vi "nominal dataset create.vi"(7 "out_dataset":i32, 8 "error in (no error)":errorcluster, 9 "description":string, 10 "name":string, 11 "client":i32) -> (0 "error out":errorcluster, 3 "function return":i32, 5 "out_dataset out":i32)   [LabVIEW 2020, in "client.lvlib"]
doc: "int32_t nominal_dataset_create(int32_t client,\n const char *name,\n const char *description,\n int32_t *out_dataset);"
uses:
  client.lvlib
  bin/nominalClient_64.dll
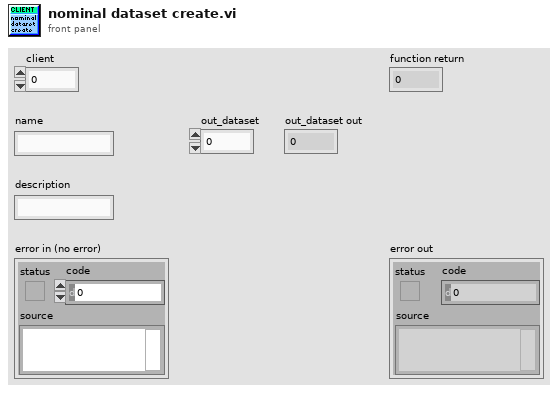
[diagram p1: front panel]
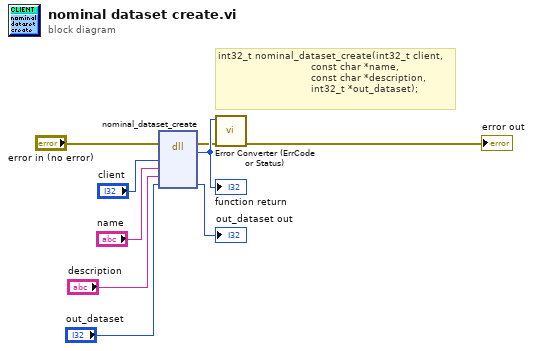
[diagram p0: block diagram]
diagram:
  # "int32_t nominal_dataset_create(int32_t client,\n                               const char *name,\n                               const char *description,\n                               int32_t *out_dataset);"
  n1 = dll-call lib="C:/code/labview-client-rs/lv_src/bin/nominalClient_*.*" fn="nominal_dataset_create"(error in="error in (no error)", "client"="client", "name"="name", "description"="description", "out_dataset"="out_dataset") -> (error out=w2:errorcluster, w9:i32, "out_dataset"=→"out_dataset out":i32)  [unwired: 5 in, 1 out]
  "function return" <- w9
  n2 = call "Error Converter (ErrCode or Status).vi"("error in (no error)"=w2, "error code"=w9) -> ("error out"=→"error out":errorcluster)  [unwired: 9 in]
